vi "oax_Generate OAT Simulated Signals.vi"(4 "noise level":dbl=0.01, 6 "add noise?":bool=TRUE, 7 "reset?":bool=TRUE, 8 "error in (no error)":errorcluster, 9 "sampling info":T2={"sampling frequency"=51200.0, "total duration [s]"=10.0} {"sampling frequency" format="%#_6p"}, 10 "ordercomponents":T1(array[cluster])=[{"order"=1.0, "amplitude"=1.0, "phase (deg)"=0.0, "order envelop"=0}, {"order"=2.0, "amplitude"=0.5, "phase (deg)"=0.0, "order envelop"=2}, {"order"=3.0, "amplitude"=0.25, "phase (deg)"=0.0, "order envelop"=1}, {"order"=10.0, "amplitude"=1.0, "phase (deg)"=0.0, "order envelop"=2}] {"order envelop" items=["None", "Sine", "Triangle"]}, 11 "signal rotating speed":u16(ring) items=["3000 RPM", "1000-6000 RPM", "6000-1000 RPM", "1000-6000-1000 RPM"]) -> (0 "error out":errorcluster, 1 "pulse/revolution":i32=1, 2 "Tach Signal":waveform(dbl), 3 "Vibration Signal":waveform(dbl))   [LabVIEW 2017]
doc: "Simulate a signal with the specified sampling and order characteristics."
uses:
  <vilib>/measure/NI_MABase.lvlib
panel:
  in  "Vibration Signal 2":waveform(dbl)={"t0"=timestamp(0 s since 1904-01-01), "dt"=0.0, "Y"=[]}
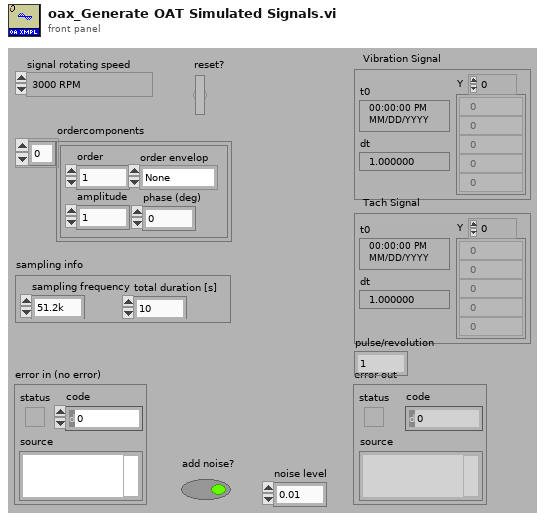
[diagram p1: front panel]
types:
  T1 = cluster{"order":dbl, "amplitude":dbl, "phase (deg)":dbl, "order envelop":u16}[]
  T2 = cluster{"sampling frequency":dbl, "total duration [s]":dbl}
  T3 = cluster{"order":dbl, "phase (deg)":dbl, "order envelop":u16, cluster{dbl, "amplitude":dbl, dbl}}
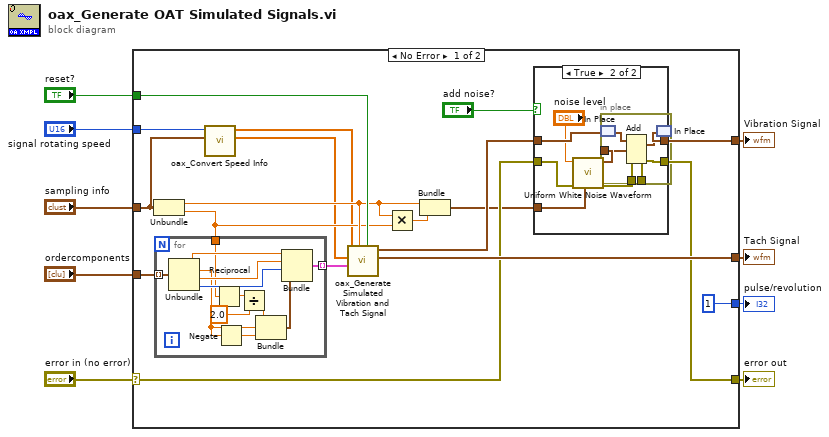
[diagram p0: block diagram]
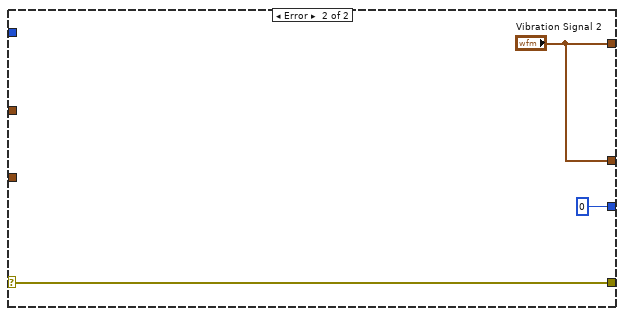
[diagram p3: hidden frame]
diagram:
  n1 = case shown="No Error" "error in (no error)" {
    selector: "error in (no error)" -> [w21 w57]
    tunnel: [w20 w57] -> w8
    tunnel: "signal rotating speed" -> [w14 _]
    tunnel: "sampling info" -> [w13 _]
    tunnel: "reset?" -> [w27 _]
    tunnel: "ordercomponents" -> [w26 _]
    tunnel: [w24 "Vibration Signal 2"] -> w3
    tunnel: [w19 "Vibration Signal 2"] -> w2
    tunnel: [1 ("pulse/revolution") 0 ("pulse/revolution")] -> w1
    frame No Error {
      n2 = Unbundle(w13) -> ("sampling frequency"=w18:dbl, "total duration [s]"=w17:dbl)
      n3 = for {
        tunnel: w26 -> [w54] mode=indexing
        tunnel: w17 -> [w50]
        tunnel: [w46] -> w25 mode=indexing
        n4 = Unbundle(w54) -> ("order"=w53:dbl, "amplitude"=w49:dbl, "phase (deg)"=w52:dbl, "order envelop"=w51:u16)
        n5 = Reciprocal(x=w50) -> (1/x=w45:dbl)
        n6 = Negate(x=w49) -> (-x=w48:dbl)
        n7 = Divide(x=w45, y=2.0) -> (x/y=w43:dbl)
        n8 = Bundle(w43, "amplitude"=w49, w48) -> (w47:cluster{dbl, "amplitude":dbl, dbl})  [unwired: 1 in]
        n9 = Bundle("order"=w53, "phase (deg)"=w52, "order envelop"=w51, w47) -> (w46:T3)  [unwired: 1 in]
      }
      n10 = call <vilib>:"oax_Convert Speed Info.vi"("sampling info"=w13, "signal rotating speed"=w14) -> ("time period"=w11:dbl[], "speed"=w12:dbl[])  [unwired: 8 in]
      n11 = call <vilib>:"oax_Generate Simulated Vibration and Tach Signal.vi"("reset?"=w27, "fs"=w18, "order info"=w25, "time period"=w11, "speed"=w12) -> ("Tach Signal"=w24:waveform(dbl), "Vibration Signal"=w22:waveform(dbl))  [unwired: 5 in]
      n12 = Multiply(x=w18, y=w17) -> (x*y=w16:dbl)
      n13 = Bundle("sampling frequency"=w18, w16) -> (w15:cluster{"sampling frequency":dbl, dbl})  [unwired: 1 in]
      n14 = case shown="True" "add noise?" {
        tunnel: w15 -> [_ w37]
        tunnel: w22 -> [w29 w36]
        tunnel: [w28 w34] -> w20
        tunnel: [w29 w33] -> w19
        tunnel: w21 -> [w28 w31]
        frame False {
        }
        frame True {
          n15 = call <vilib>:"Uniform White Noise Waveform.vi"("sampling info"=w37, "error in (no error)"=w31, "amplitude"="noise level") -> ("error out"=w35:errorcluster, "signal out"=w32:waveform(dbl))  [unwired: 7 in]
          n16 = in-place {
            in-place-border: w35 -> [w41]
            in-place-border: [w40] -> w34
            in-place-border: w32 -> [w38]
            n17 = in-place-match #1(w36) -> (w42:waveform(dbl))
            n18 = Add(1:w38, 2:w42, 4:w41) -> (0:w39:waveform(dbl), 3:w40:errorcluster)
            n19 = in-place-match #1(w39) -> (w33:waveform(dbl))
          }
        }
      }
    }
    frame Error {
    }
  }
  "error out" <- w8
  "Vibration Signal" <- w2
  "Tach Signal" <- w3
  "pulse/revolution" <- w1
